vi "FTW-Example-SLASD-Connect.vi"(0 "IP Address":string, 9 "Timeout":i32=1000 format="%dmsec", 11 "error in":errorcluster) -> (4 "FTW Actor Connector":refnum<class "FTW-Example-SLASD.lvclass">, 6 "Subscription Registration Refnum":refnum<event-registration>, 15 "error out":errorcluster)   [LabVIEW 2013, in "FTW-Example-SLASD.lvclass"]
uses:
  FTW-Example-SLASD.lvclass
  Actor/src/Message/Base/FTW-Message.lvclass
  FTW-Example-SLASD.lvclass/FTW-Example-SLASD.ctl
  Actor/src/Subscriber/FTW-Subscriber.lvclass
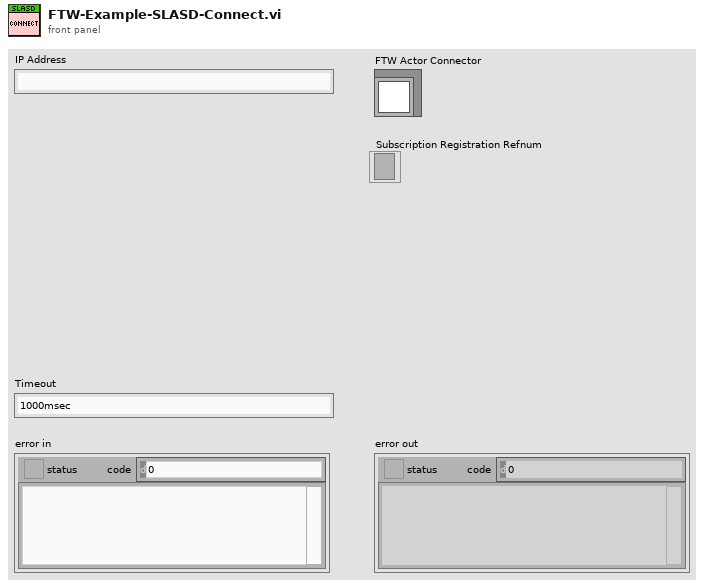
[diagram p1: front panel]
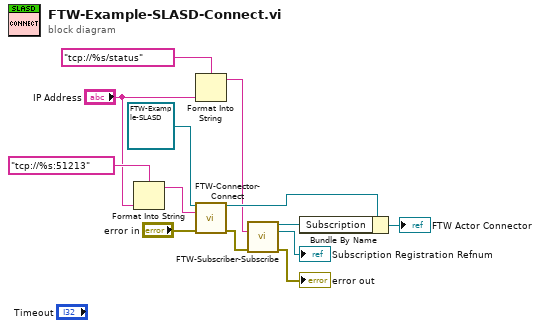
[diagram p0: block diagram]
diagram:
  n1 = Format Into String(format string="tcp://%s:51213" ("Configuration"), "IP Address") -> (resulting string=w8:string)  [unwired: 2 in, 1 out]
  n2 = Format Into String(format string="tcp://%s/status" ("Configuration"), "IP Address") -> (resulting string=w3:string)  [unwired: 2 in, 1 out]
  n3 = call-dynamic "FTW-Connector-Connect.vi"("FTW Actor Connector Type"=refnum<class "FTW-Example-SLASD.lvclass"> refnum ("TTK_Splashscreen.lvclass"), "Instance Inbox Address"=w8, "error in"="error in") -> ("FTW Actor Connector"=w11:refnum<class "FTW-Example-SLASD.lvclass">, "error out"=w12:errorcluster)  [unwired: 11 in]
  n4 = call "FTW-Subscriber-Subscribe.vi"("Addresses"=w3, "error in"=w12) -> ("FTW-Subscription Out"=w2:refnum<class "FTW-Subscriber.lvclass">, "Subscriber Registration"=→"Subscription Registration Refnum":refnum<event-registration>, "error out"=→"error out":errorcluster)  [unwired: 11 in]
  n5 = Bundle By Name(cluster=w11, "Subscription"=w2) -> (→"FTW Actor Connector":refnum<class "FTW-Example-SLASD.lvclass">)
